vi "Initialize Laser.vi"(11 "VISA Refnum in":refnum<visa-resource-name>="USB0::0x1313::0x804F::M00445403::INSTR" caption="resource name") -> (0 "error out":errorcluster {"code" format="%.0x"})   [LabVIEW 2012]
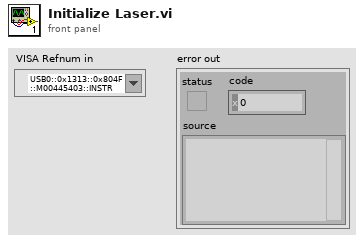
[diagram p1: front panel]
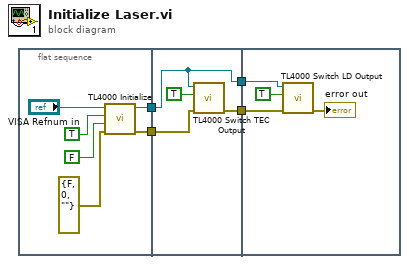
[diagram p0: block diagram]
diagram:
  n1 = flat-sequence {
    tunnel: [w8] -> w4
    tunnel: [w6] -> w3
    tunnel: w4 -> [w12]
    tunnel: w3 -> [w13]
    tunnel: [w12] -> w2
    tunnel: [w11] -> w1
    tunnel: w2 -> [w16]
    tunnel: w1 -> [w15]
    frame #0 {
      n2 = call <instrlib>:"TL4000 Initialize.vi"("error in (no error)"=errorcluster {"status"=FALSE, "code"=0, "source"=""}, "Reset Device (Reset Device)"=FALSE, "ID Query (Do Query)"=TRUE, "resource name"="VISA Refnum in") -> ("error out"=w6:errorcluster, "instrument handle out"=w8:refnum<visa-resource-name>)  [unwired: 6 in]
    }
    frame #1 {
      n3 = call <instrlib>:"TL4000 Switch TEC Output.vi"("error in (no error)"=w13, "TEC Output (Off)"=TRUE, "instrument handle"=w12) -> ("error out"=w11:errorcluster)  [unwired: 7 in, 1 out]
    }
    frame #2 {
      n4 = call <instrlib>:"TL4000 Switch LD Output.vi"("error in (no error)"=w15, "LD Output (Off)"=TRUE, "instrument handle"=w16) -> ("error out"=→"error out":errorcluster)  [unwired: 7 in, 1 out]
    }
  }
